vi "DAQmx Create Channel (CI-Pulse Width).vi"(0 "task in":refnum<k21>, 1 "maximum value":dbl=0.1 format="%.6f", 2 "minimum value":dbl=1e-06 format="%.6f", 5 "counter":tag, 7 "name to assign":string, 9 "units":i32(ring)=10364 items=["Seconds"=10364, "Ticks"=10304, "From Custom Scale"=10065], 11 "error in":errorcluster, 12 "custom scale name":tag, 13 "starting edge":i32(ring)=10280 items=["Rising"=10280, "Falling"=10171]) -> (4 "task out":refnum<k21>, 15 "error out":errorcluster)   [LabVIEW 2018]
doc: "Creates a channel to measure the width of a digital pulse. <B>starting edge</B> determines whether to measure a high pulse or low pulse. With the exception of devices that support multi-counter tasks, you can create only one counter input channel at a time with this VI because a task can contain only one counter input channel. To read from multiple counters simultaneously, use a separate task for each counter. Connect the input signal to the default input terminal of the counter unless you select a different input terminal."
uses:
  nilvaiu.dll
panel:
  # "input limits"
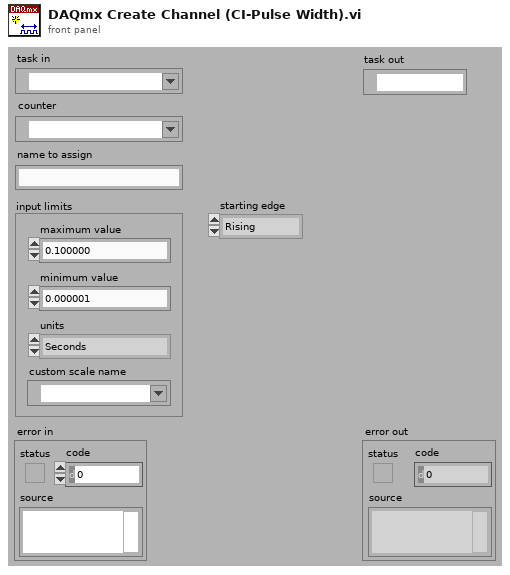
[diagram p1: front panel]
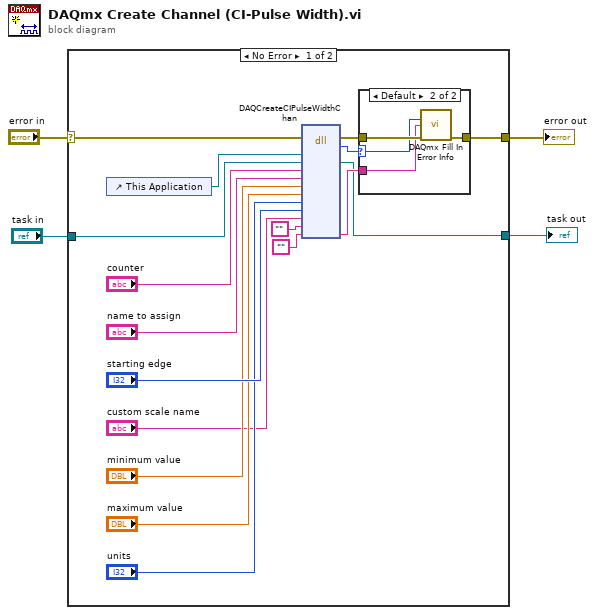
[diagram p0: block diagram]
diagram:
  n1 = case shown="No Error" "error in" {
    selector: "error in" -> [w6 w28]
    tunnel: [w9 w28] -> w4
    tunnel: "task in" -> [w8 w27]
    tunnel: [w7 w27] -> w2
    frame No Error {
      n2 = control-ref of="This Application"() -> (w18:refnum<vi>)
      n3 = dll-call lib="nilvaiu.*" fn="DAQCreateCIPulseWidthChan"(error in=w6, "lvAppRef"=w18, "refObjPtr"=w8, "counter"="counter", "channelNameIn"="name to assign", "minVal"="minimum value", "maxVal"="maximum value", "units"="units", "startingEdge"="starting edge", "customScaleName"="custom scale name", "channelNamesOut"="", "extendedErrorInfo"="") -> (error out=w21:errorcluster, "return type"=w20:i32, "refObjPtr"=w7:refnum<k21>, "extendedErrorInfo"=w19:string)  [unwired: 11 in, 1 out]
      n4 = case shown="Default" w20 {
        selector: w20 -> [_ w24]
        tunnel: w21 -> [w22 w26]
        tunnel: [w22 w25] -> w9
        tunnel: w19 -> [_ w23]
        frame 0 {
        }
        frame Default {
          n5 = call "DAQmx Fill In Error Info.vi"("status code"=w24, "extended error info"=w23, "error in"=w26) -> ("error out"=w25:errorcluster)  [unwired: 1 in, 11 out]
        }
      }
    }
    frame Error {
    }
  }
  "error out" <- w4
  "task out" <- w2
